vi "ASPftpSummary.vi"() -> ()   [LabVIEW 2012]
uses:
  <vilib>/addons/database/Auxilliary.llb/DB Tools Cursor Type.ctl
  <vilib>/addons/database/Connection.llb/DB Tools Open Connec (Path).vi
  <vilib>/addons/database/Connection.llb/Conn Execute.vi
  <vilib>/addons/database/Recordset.llb/Rec Fetch Recordset Data (R).vi
  <vilib>/addons/database/Recordset.llb/Rec Destroy - Connection.vi
  <vilib>/addons/database/Recordset.llb/Rec Fetch Integer Data (R).vi
  <vilib>/addons/database/Recordset.llb/Rec Fetch String Data (R).vi
  <vilib>/addons/database/_DB Variant To Data/Database Variant To Data.xnode
  <vilib>/addons/database/NI_Database_API.lvlib
panel:
  out "spreadsheet string":string
  out "array":string[][](array[string])
  out "error out":errorcluster
  out "data 2":i32
  out "data 3":string
  out "data 4":i32
  out "data":string
  out "concatenated string":string
  out "String":string
  out "error out 3":errorcluster
  out "error out 2":errorcluster
  out "concatenated string 2":string
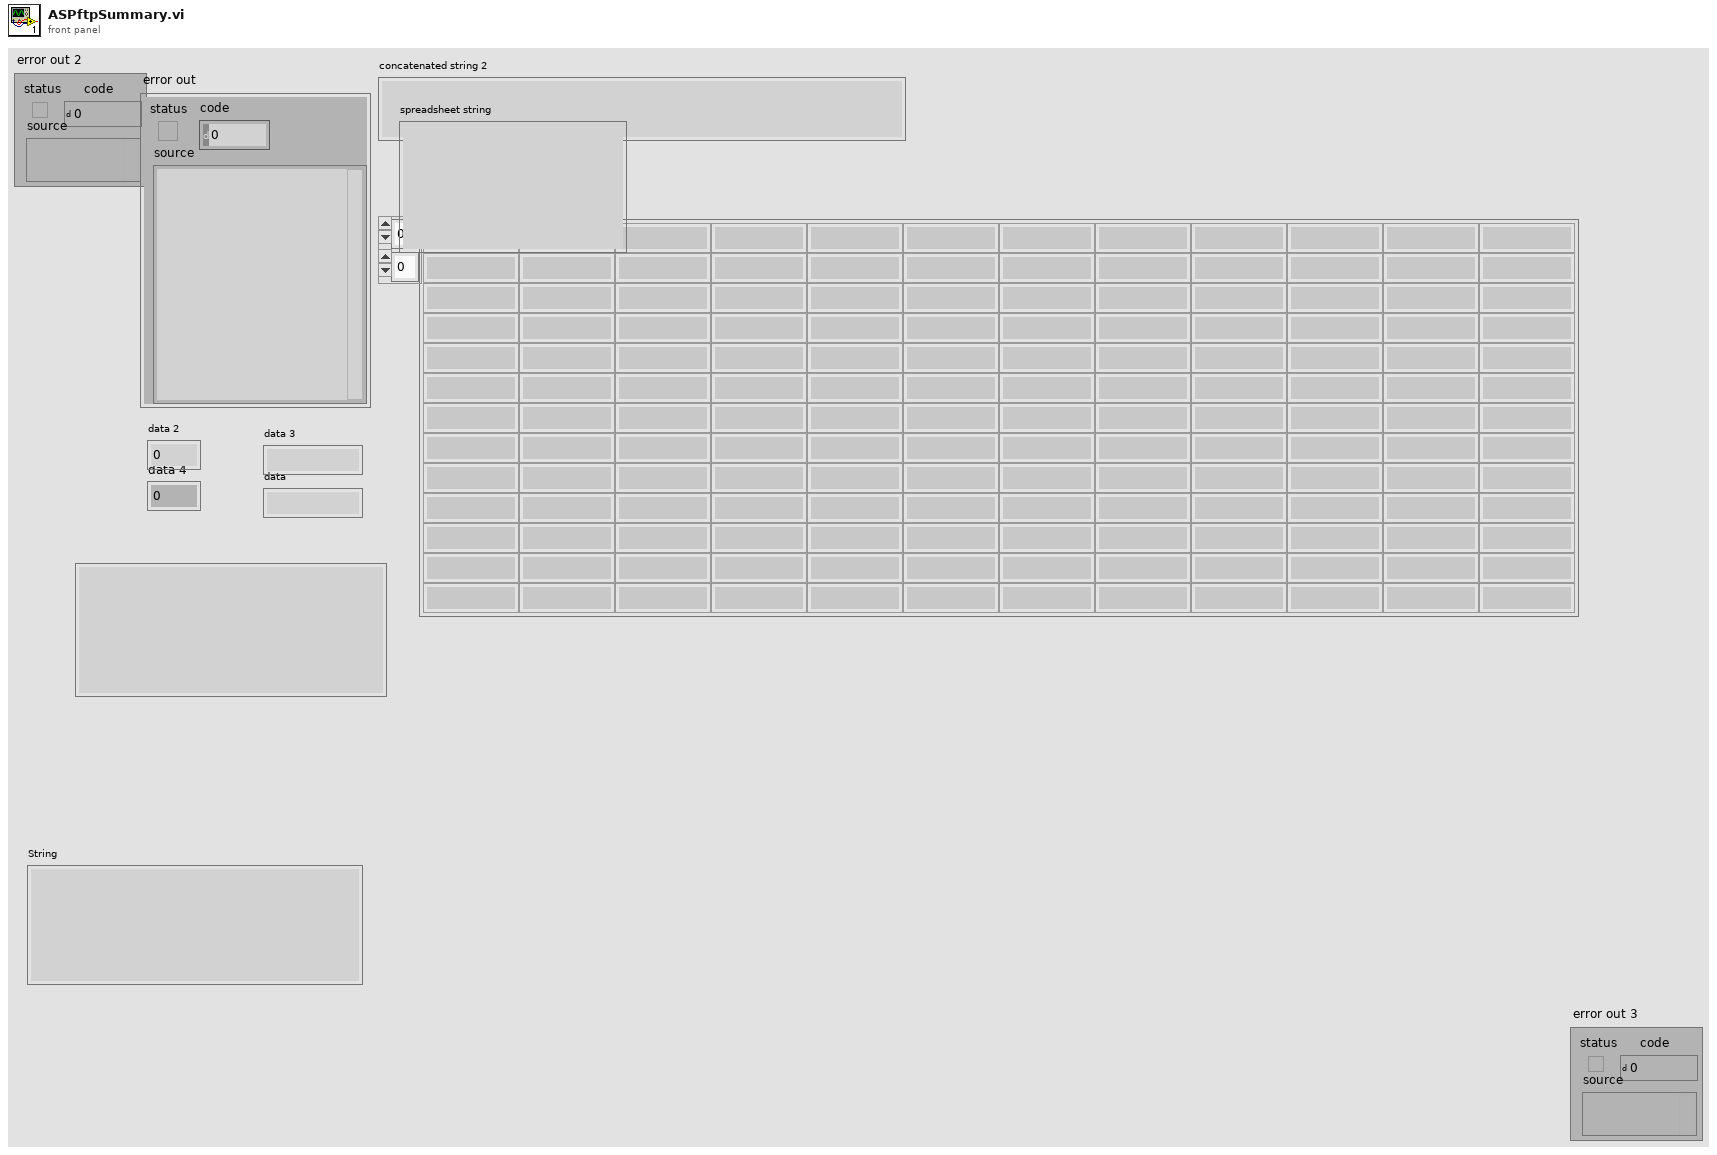
[diagram p1: front panel]
types:
  T1 = typedef "NI_Database_API.lvlib/DB Tools Cursor Type.ctl" = enum16{"forward-only", "keyset", "dynamic", "static"}
  T2 = typedef "NI_Database_API.lvlib/Conn ObjectReference.ctl" = refnum<k1>
  T3 = typedef "NI_Database_API.lvlib/Rec ObjectReference.ctl" = refnum<k1>
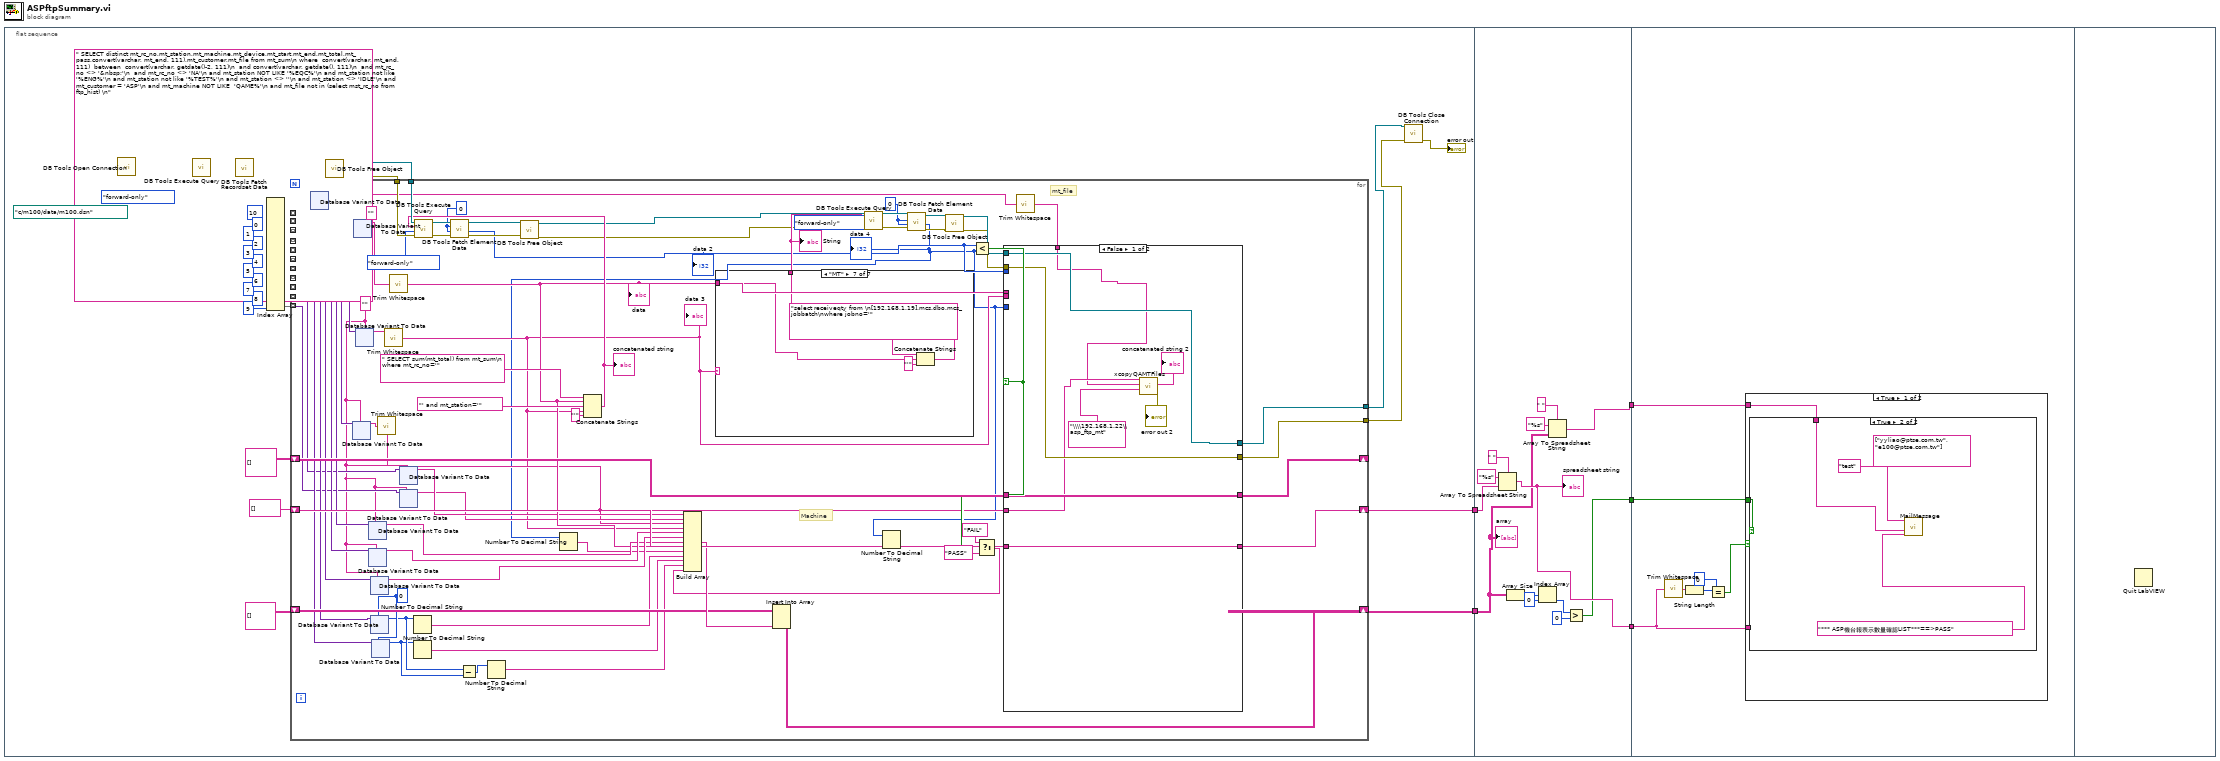
[diagram p0: block diagram]
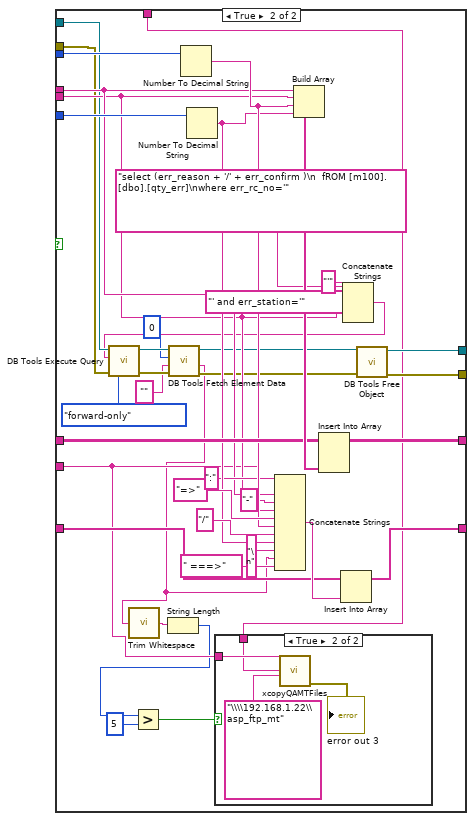
[diagram p2: hidden frame]
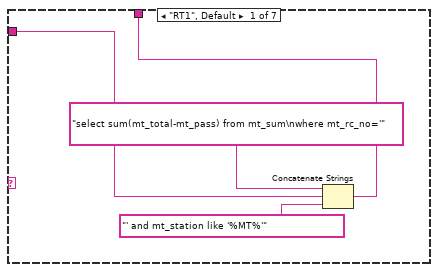
[diagram p4: hidden frame]
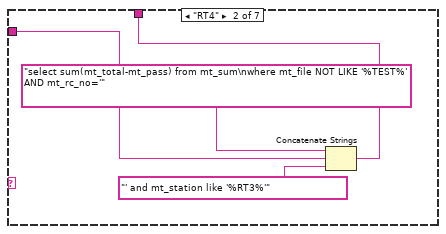
[diagram p5: hidden frame]
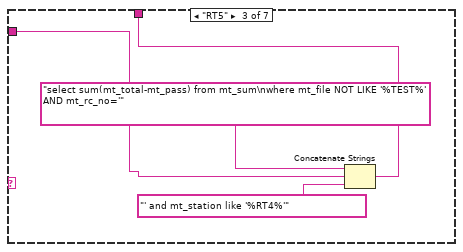
[diagram p6: hidden frame]
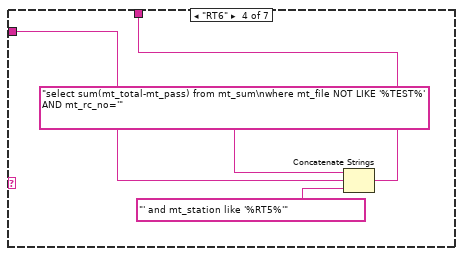
[diagram p7: hidden frame]
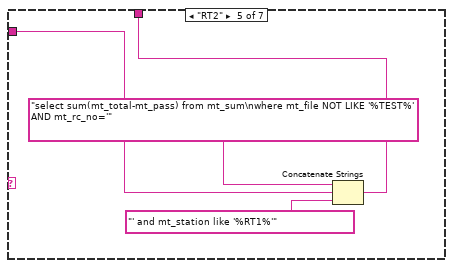
[diagram p8: hidden frame]
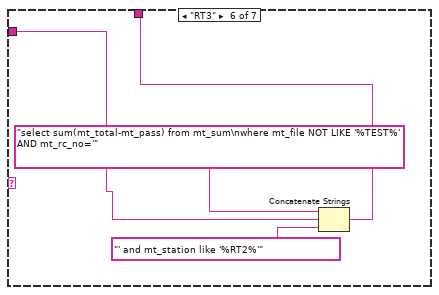
[diagram p9: hidden frame]
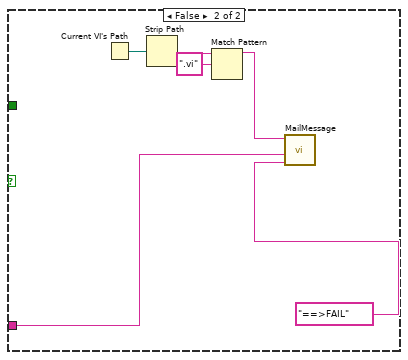
[diagram p11: hidden frame]
diagram:
  n1 = flat-sequence {
    tunnel: [w28] -> w5
    tunnel: [w24] -> w4
    tunnel: w5 -> [w563]
    tunnel: w4 -> [w558]
    tunnel: [w562] -> w3
    tunnel: [w559] -> w2
    tunnel: [w553] -> w1
    tunnel: w3 -> [w572]
    tunnel: w2 -> [w567]
    tunnel: w1 -> [w566]
    frame #0 {
      n2 = call-poly <vilib>:"DB Tools Open Connection.vi"("connection information"=path "c:/m100/data/m100.dsn") -> ("error out"=w45:errorcluster, "connection reference"=w46:T2)  [unwired: 7 in]
      n3 = call-poly <vilib>:"DB Tools Execute Query.vi"("error in (no error)"=w45, "cursor type"=DB_Tools_Cursor_Type."forward-only", "SQL query"=" SELECT distinct mt_rc_no,mt_station,mt_machine,mt_device,mt_start,mt_end,mt_total,mt_pass,convert(varchar, mt_end, 111),mt_customer,mt_file from mt_sum\n where  convert(varchar, mt_end, 111)  between  convert(varchar, getdate()-2, 111)\n  and convert(varchar, getdate(), 111)\n  and mt_rc_no <> '&nbsp;'\n  and mt_rc_no <> 'NA'\n and mt_station NOT LIKE '%EQC%'\n and mt_station not like '%ENG%'\n and mt_station not like '%TEST%'\n and mt_station <> ''\n and mt_station <> 'IDLE'\n and mt_customer = 'ASP'\n and mt_machine NOT LIKE  'QAME%'\n and mt_file not in (select mst_rc_no from ftp_hist) \n", "connection reference"=w46) -> ("error out"=w43:errorcluster, "recordset reference"=w44:T3)  [unwired: 4 in]
      n4 = call-poly <vilib>:"DB Tools Fetch Recordset Data.vi"("error in (no error)"=w43, "recordset reference"=w44) -> ("error out"=w41:errorcluster, "recordset data"=w37:variant[][], "recordset reference out"=w42:T3)  [unwired: 3 in]
      n5 = Index Array(array=w37, index (col) #1=10 ("disabled index (col)"), index (col) #2=0 ("disabled index (col)"), index (col) #3=1 ("index (col)"), index (col) #4=2 ("index (col)"), index (col) #5=3 ("index (col)"), index (col) #6=4 ("index (col)"), index (col) #7=5 ("index (col)"), index (col) #8=6 ("index (col)"), index (col) #9=7 ("index (col)"), index (col) #10=8 ("index (col)"), index (col) #11=9 ("index (col)")) -> (element #1=w6:variant[], element #2=w36:variant[], element #3=w33:variant[], element #4=w26:variant[], element #5=w20:variant[], element #6=w19:variant[], element #7=w18:variant[], element #8=w15:variant[], element #9=w14:variant[], element #10=w11:variant[], element #11=w10:variant[])  [unwired: 11 in]
      n6 = call-poly <vilib>:"DB Tools Free Object.vi"("error in (no error)"=w41, "recordset reference"=w42) -> ("error out"=w31:errorcluster, "connection reference"=w32:T2)  [unwired: 8 in]
      n7 = for {
        tunnel: w36 -> [w111] mode=indexing
        tunnel: w33 -> [w119] mode=indexing
        tunnel: w32 -> [w110]
        tunnel: w31 -> [w109]
        shift-right: [w94] -> _
        shift-left: string[][] [] ("array") -> [w93]
        shift-right: [w55] -> w28
        shift-left: string[] [] ("array") -> [w92]
        tunnel: w26 -> [w91] mode=indexing
        shift-right: [w85] -> w24
        shift-left: string[][] [] ("array") -> [w83]
        tunnel: w20 -> [w82] mode=indexing
        tunnel: w19 -> [w81] mode=indexing
        tunnel: w18 -> [w80] mode=indexing
        tunnel: w15 -> [w79] mode=indexing
        tunnel: w14 -> [w78] mode=indexing
        tunnel: w11 -> [w73] mode=indexing
        tunnel: w10 -> [w72] mode=indexing
        tunnel: [w60] -> w9
        tunnel: [w48] -> w8
        tunnel: w6 -> [w59] mode=indexing
        w77 = 0
        w112 = 0
        w101 = 0
        w71 = ""
        w58 = ""
        # "Machine"
        # "mt_file"
        n8 = xnode "Database Variant To Data"("database variant"=w59, "type"=w58) -> ("data"=w57:string)  [unwired: 1 in, 1 out]
        n9 = xnode "Database Variant To Data"("database variant"=w91, "type"=w71) -> ("data"=w90:string)  [unwired: 1 in, 1 out]
        n10 = xnode "Database Variant To Data"("database variant"=w111, "type"=w58) -> ("data"=w95:string)  [unwired: 1 in, 1 out]
        n11 = xnode "Database Variant To Data"("database variant"=w119, "type"=w71) -> ("data"=w96:string)  [unwired: 1 in, 1 out]
        n12 = xnode "Database Variant To Data"("database variant"=w82, "type"=w71) -> ("data"=w68:string)  [unwired: 1 in, 1 out]
        n13 = xnode "Database Variant To Data"("database variant"=w81, "type"=w71) -> ("data"=w70:string)  [unwired: 1 in, 1 out]
        n14 = xnode "Database Variant To Data"("database variant"=w80, "type"=w71) -> ("data"=w69:string)  [unwired: 1 in, 1 out]
        n15 = xnode "Database Variant To Data"("database variant"=w79, "type"=w77) -> ("data"=w76:i32)  [unwired: 1 in, 1 out]
        n16 = xnode "Database Variant To Data"("database variant"=w78, "type"=w77) -> ("data"=w75:i32)  [unwired: 1 in, 1 out]
        n17 = call <vilib>:"Trim Whitespace.vi"("string"=w90) -> ("trimmed string"=w64:string)  [unwired: 1 in]
        n18 = call <vilib>:"Trim Whitespace.vi"("string"=w96) -> ("trimmed string"=w63:string)  [unwired: 1 in]
        "data 3" <- w63
        n19 = call <vilib>:"Trim Whitespace.vi"("string"=w95) -> ("trimmed string"=w67:string)  [unwired: 1 in]
        "data" <- w67
        n20 = xnode "Database Variant To Data"("database variant"=w72, "type"=w71) -> ("data"=w65:string)  [unwired: 1 in, 1 out]
        n21 = xnode "Database Variant To Data"("database variant"=w73, "type"=w71) -> ("data"=w66:string)  [unwired: 1 in, 1 out]
        n22 = Number To Decimal String(number=w76) -> (decimal integer string=w51:string)  [unwired: 1 in]
        n23 = Number To Decimal String(number=w75) -> (decimal integer string=w52:string)  [unwired: 1 in]
        n24 = Subtract(x=w76, y=w75) -> (x-y=w74:i32)
        n25 = Number To Decimal String(number=w74) -> (decimal integer string=w53:string)  [unwired: 1 in]
        n26 = Concatenate Strings(" SELECT sum(mt_total) from mt_sum\n where mt_rc_no='", w67, "' and mt_station='" ("string"), w63, "'" ("string")) -> (w102:string)
        "concatenated string" <- w102
        n27 = call-poly <vilib>:"DB Tools Execute Query.vi"("error in (no error)"=w109, "cursor type"=DB_Tools_Cursor_Type."forward-only", "SQL query"=w102, "connection reference"=w110) -> ("error out"=w107:errorcluster, "recordset reference"=w108:T3)  [unwired: 4 in]
        n28 = call-poly <vilib>:"DB Tools Fetch Element Data.vi"("error in (no error)"=w107, "type"=w101, "column index"=w101, "recordset reference"=w108) -> ("error out"=w99:errorcluster, "data"=w89:i32, "recordset reference out"=w100:T3)  [unwired: 3 in]
        "data 2" <- w89
        n29 = call-poly <vilib>:"DB Tools Free Object.vi"("error in (no error)"=w99, "recordset reference"=w100) -> ("error out"=w98:errorcluster, "connection reference"=w97:T2)  [unwired: 8 in]
        n30 = case shown="\"MT\"" w63 {
          tunnel: w67 -> [w462 w465 w469 w473 w478 w481 w487]
          tunnel: [w461 w466 w470 w474 w477 w482 w486] -> w114
          frame "RT1", Default {
            n31 = Concatenate Strings("select sum(mt_total-mt_pass) from mt_sum\nwhere mt_rc_no='" ("string"), w462, "' and mt_station like '%MT%'" ("string")) -> (w461:string)
          }
          frame "RT4" {
            n32 = Concatenate Strings("select sum(mt_total-mt_pass) from mt_sum\nwhere mt_file NOT LIKE '%TEST%' AND mt_rc_no='" ("string"), w465, "' and mt_station like '%RT3%'" ("string")) -> (w466:string)
          }
          frame "RT5" {
            n33 = Concatenate Strings("select sum(mt_total-mt_pass) from mt_sum\nwhere mt_file NOT LIKE '%TEST%' AND mt_rc_no='" ("string"), w469, "' and mt_station like '%RT4%'" ("string")) -> (w470:string)
          }
          frame "RT6" {
            n34 = Concatenate Strings("select sum(mt_total-mt_pass) from mt_sum\nwhere mt_file NOT LIKE '%TEST%' AND mt_rc_no='" ("string"), w473, "' and mt_station like '%RT5%'" ("string")) -> (w474:string)
          }
          frame "RT2" {
            n35 = Concatenate Strings("select sum(mt_total-mt_pass) from mt_sum\nwhere mt_file NOT LIKE '%TEST%' AND mt_rc_no='" ("string"), w478, "' and mt_station like '%RT1%'" ("string")) -> (w477:string)
          }
          frame "RT3" {
            n36 = Concatenate Strings("select sum(mt_total-mt_pass) from mt_sum\nwhere mt_file NOT LIKE '%TEST%' AND mt_rc_no='" ("string"), w481, "' and mt_station like '%RT2%'" ("string")) -> (w482:string)
          }
          frame "MT" {
            n37 = Concatenate Strings("select receiveqty from \n[192.168.1.19].mcs.dbo.mcs_jobbatch\nwhere jobno='" ("string"), w487, "'" ("string")) -> (w486:string)
          }
        }
        "String" <- w114
        n38 = call-poly <vilib>:"DB Tools Execute Query.vi"("error in (no error)"=w98, "cursor type"=DB_Tools_Cursor_Type."forward-only", "SQL query"=w114, "connection reference"=w97) -> ("error out"=w113:errorcluster, "recordset reference"=w117:T3)  [unwired: 4 in]
        n39 = call-poly <vilib>:"DB Tools Fetch Element Data.vi"("error in (no error)"=w113, "type"=w112, "column index"=w112, "recordset reference"=w117) -> ("error out"=w115:errorcluster, "data"=w50:i32, "recordset reference out"=w116:T3)  [unwired: 3 in]
        "data 4" <- w50
        n40 = Number To Decimal String(number=w50) -> (decimal integer string=w49:string)  [unwired: 1 in]
        n41 = Number To Decimal String(number=w50) -> ()  [unwired: 1 in, 1 out]
        n42 = call-poly <vilib>:"DB Tools Free Object.vi"("error in (no error)"=w115, "recordset reference"=w116) -> ("error out"=w61:errorcluster, "connection reference"=w62:T2)  [unwired: 8 in]
        n43 = Less?(x=w89, y=w50) -> (x < y?=w88:bool)
        n44 = Select(t="FAIL", s=w88, f="PASS") -> (s? t:f=w54:string)
        n45 = Build Array(w66, w65, w64, w63, w70, w69, w68, w67, w49, w51, w52, w53, w54) -> (w84:string[])
        n46 = Insert Into Array(array=w83, new element=w84) -> (w85:string[][])  [unwired: 2 in]
        n47 = call <vilib>:"Trim Whitespace.vi"("string"=w57) -> ("trimmed string"=w56:string)  [unwired: 1 in]
        n48 = case shown="False" w88 {
          tunnel: w67 -> [_ w441]
          tunnel: w63 -> [_ w439]
          tunnel: w89 -> [_ w456]
          tunnel: w50 -> [_ w455]
          tunnel: [w416 w453] -> w94
          tunnel: w93 -> [w416 w452]
          tunnel: [w415 w446] -> w55
          tunnel: w92 -> [w415 w445]
          tunnel: w64 -> [w412 w423]
          tunnel: w62 -> [w414 w433]
          tunnel: w61 -> [w413 w432]
          tunnel: [w414 w425] -> w60
          tunnel: [w413 w424] -> w48
          tunnel: w56 -> [w410 w422]
          frame False {
            n49 = call "xcopyQAMTFiles.vi"("Destination"="\\\\192.168.1.22\\asp_ftp_mt", "SourceFile"=w410, "Machine"=w412) -> ("error out"=→"error out 2":errorcluster, "concatenated string"=→"concatenated string 2":string)  [unwired: 6 in]
          }
          frame True {
            n50 = Number To Decimal String(number=w456) -> (decimal integer string=w450:string)  [unwired: 1 in]
            n51 = Number To Decimal String(number=w455) -> (decimal integer string=w448:string)  [unwired: 1 in]
            n52 = Build Array(w441, w439, w450, w448) -> (w454:string[])
            n53 = Insert Into Array(array=w452, new element=w454) -> (w453:string[][])  [unwired: 2 in]
            n54 = Concatenate Strings("select (err_reason + '/' + err_confirm )\n  fROM [m100].[dbo].[qty_err]\nwhere err_rc_no='" ("string"), w441, "' and err_station='" ("string"), w439, "'" ("string")) -> (w430:string)
            n55 = call-poly <vilib>:"DB Tools Execute Query.vi"("error in (no error)"=w432, "cursor type"=DB_Tools_Cursor_Type."forward-only", "SQL query"=w430, "connection reference"=w433) -> ("error out"=w437:errorcluster, "recordset reference"=w436:T3)  [unwired: 4 in]
            n56 = call-poly <vilib>:"DB Tools Fetch Element Data.vi"("error in (no error)"=w437, "type"="", "column index"=0, "recordset reference"=w436) -> ("error out"=w434:errorcluster, "data"=w420:string, "recordset reference out"=w435:T3)  [unwired: 3 in]
            n57 = call <vilib>:"Trim Whitespace.vi"("string"=w420) -> ("trimmed string"=w421:string)  [unwired: 1 in]
            n58 = String Length(string=w421) -> (length=w419:i32)
            n59 = Greater?(x=w419, y=5) -> (0:w417:bool)
            n60 = case shown="True" w417 {
              tunnel: w423 -> [_ w458]
              tunnel: w422 -> [_ w457]
              frame False {
              }
              frame True {
                n61 = call "xcopyQAMTFiles.vi"("Destination"="\\\\192.168.1.22\\asp_ftp_mt", "SourceFile"=w457, "Machine"=w458) -> ("error out"=→"error out 3":errorcluster)  [unwired: 6 in, 1 out]
              }
            }
            n62 = Concatenate Strings(w423, ":" ("string"), w441, "-" ("string"), w439, "=>" ("string"), w450, "/" ("string"), w448, " ===>" ("string"), w420, "\n" ("string")) -> (w447:string)
            n63 = Insert Into Array(array=w445, new element=w447) -> (w446:string[])  [unwired: 1 in]
            n64 = call-poly <vilib>:"DB Tools Free Object.vi"("error in (no error)"=w434, "recordset reference"=w435) -> ("error out"=w424:errorcluster, "connection reference"=w425:T2)  [unwired: 8 in]
          }
        }
      }
      n65 = call <vilib>:"DB Tools Close Connection.vi"("error in (no error)"=w8, "connection reference"=w9) -> ("error out"=→"error out":errorcluster)  [unwired: 5 in]
    }
    frame #1 {
      n66 = Array To Spreadsheet String(delimiter (Tab)=" ", array=w563, 3:"%s" ("format string")) -> (spreadsheet string=w562:string)
      "spreadsheet string" <- w562
      n67 = Array Size(array=w558) -> (size(s)=w557:i32[])
      n68 = Index Array(array=w557, index=0) -> (element=w555:i32)
      n69 = Array To Spreadsheet String(delimiter (Tab)=" ", array=w558, 3:"%s" ("format string")) -> (spreadsheet string=w559:string)
      n70 = Greater?(x=w555, y=0) -> (0:w553:bool)
      "array" <- w558
    }
    frame #2 {
      n71 = call <vilib>:"Trim Whitespace.vi"("string"=w572) -> ("trimmed string"=w571:string)  [unwired: 1 in]
      n72 = String Length(string=w571) -> (length=w570:i32)
      n73 = Equal?(x=w570, y=0) -> (x = y?=w568:bool)
      n74 = case shown="True" w568 {
        tunnel: w572 -> [_ w578]
        tunnel: w567 -> [w574 _]
        tunnel: w566 -> [w573 _]
        frame True {
          n75 = case shown="True" w573 {
            tunnel: w574 -> [_ w575]
            frame False {
            }
            frame True {
              (unwired) string[] ["yyliao@ptse.com.tw", "e100@ptse.com.tw"] ("recipients")
              n76 = call "MailMessage.vi"("AddSubject"="*** ASP機台報表示數量確認LIST***==>PASS" ("subject ([No Subject])"), "message"=w575, "program"="test") -> ()  [unwired: 9 in]
            }
          }
        }
        frame False {
          n77 = Current VI's Path() -> (path=w583:path)
          n78 = Strip Path(path=w583) -> (name=w582:string)  [unwired: 1 out]
          n79 = Match Pattern(string=w582, regular expression=".vi") -> (before substring=w580:string)  [unwired: 1 in, 3 out]
          n80 = call "MailMessage.vi"("AddSubject"="==>FAIL" ("subject ([No Subject])"), "message"=w578, "program"=w580) -> ()  [unwired: 9 in]
        }
      }
    }
    frame #3 {
      n81 = Quit LabVIEW() -> ()  [unwired: 1 in]
    }
  }
